vi "Build Label Properties.vi"(8 "error in (no error)":errorcluster, 10 "Labels":T1) -> (0 "error out":errorcluster, 2 "name":string, 4 "Prop Names":string[](array[string]), 6 "Prop Values":variant[](array[variant]))   [LabVIEW 2015, in "AIT 429 System Explorer.lvlib"]
uses:
  AIT 429 System Explorer.lvlib
  Controls/AIT_Label.ctl
  Controls/AIT_Word.ctl
  Controls/ARINCParam.ctl
  Shared/Controls and Global/TransferType.ctl
  Shared/Controls and Global/Global.vi
  Shared/AIT 429 Shared.lvlib
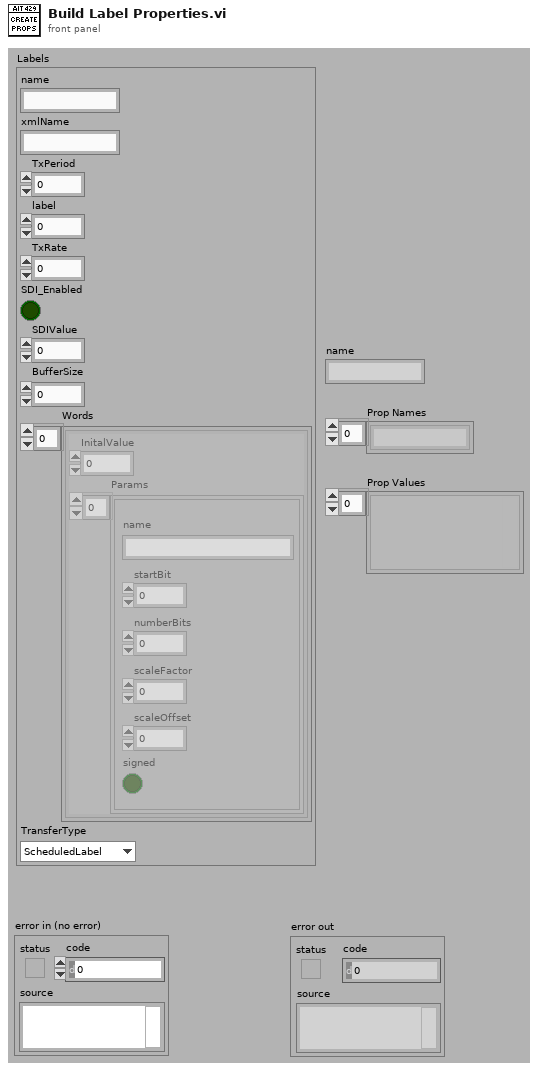
[diagram p1: front panel]
types:
  T1 = typedef "AIT 429 System Explorer.lvlib/AIT_Label.ctl" = cluster{"name":string, "xmlName":string, "TxPeriod":u32, "label":u32, "TxRate":dbl, "SDI_Enabled":bool, "SDIValue":u8, "BufferSize":u32, "Words":T2[], "TransferType":T4}
  T2 = typedef "AIT 429 System Explorer.lvlib/AIT_Word.ctl" = cluster{"InitalValue":u32, "Params":T3[]}
  T3 = typedef "AIT 429 System Explorer.lvlib/ARINCParam.ctl" = cluster{"name":string, "startBit":i32, "numberBits":i32, "scaleFactor":dbl, "scaleOffset":dbl, "signed":bool}
  T4 = typedef "AIT 429 Shared.lvlib/TransferType.ctl" = enum16{"ScheduledLabel", "Acyclic", "Block", "Strobe"}
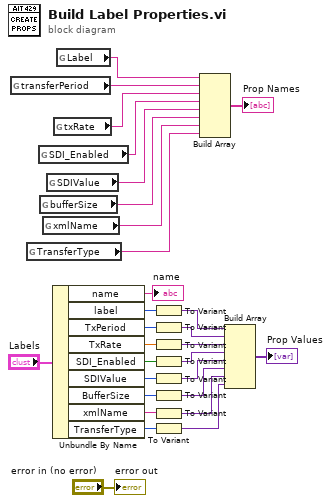
[diagram p0: block diagram]
diagram:
  n1 = global read "Global.vi" "transferPeriod"() -> (w21:string)
  n2 = global read "Global.vi" "TransferType"() -> (w7:string)
  n3 = global read "Global.vi" "SDI_Enabled"() -> (w15:string)
  n4 = global read "Global.vi" "bufferSize"() -> (w4:string)
  n5 = global read "Global.vi" "xmlName"() -> (w10:string)
  n6 = global read "Global.vi" "SDIValue"() -> (w14:string)
  n7 = Unbundle By Name("Labels") -> ("name"=→"name":string, "label"=w22:u32, "TxPeriod"=w28:u32, "TxRate"=w18:dbl, "SDI_Enabled"=w13:bool, "SDIValue"=w9:u8, "BufferSize"=w2:u32, "xmlName"=w3:string, "TransferType"=w6:T4)
  n8 = global read "Global.vi" "txRate"() -> (w16:string)
  n9 = global read "Global.vi" "Label"() -> (w20:string)
  n10 = To Variant(anything=w22) -> (Variant=w25:variant)
  n11 = To Variant(anything=w28) -> (Variant=w24:variant)
  n12 = To Variant(anything=w18) -> (Variant=w17:variant)
  n13 = To Variant(anything=w13) -> (Variant=w12:variant)
  n14 = To Variant(anything=w9) -> (Variant=w11:variant)
  n15 = To Variant(anything=w2) -> (Variant=w1:variant)
  n16 = To Variant(anything=w3) -> (Variant=w8:variant)
  n17 = To Variant(anything=w6) -> (Variant=w5:variant)
  n18 = Build Array(w20, w21, w16, w15, w14, w4, w10, w7) -> (→"Prop Names":string[])
  n19 = Build Array(w25, w24, w17, w12, w11, w1, w8, w5) -> (→"Prop Values":variant[])
  "error out" <- "error in (no error)"
